vi "Get Message.vi"(8 "error in (no error)":errorcluster, 11 "SPARC4_GUI in":refnum<class "SPARC4_GUI.lvclass">) -> (0 "error out":errorcluster, 3 "SPARC4_GUI out":refnum<class "SPARC4_GUI.lvclass">)   [LabVIEW 2018, in "SPARC4_GUI.lvclass"]
uses:
  SPARC4_GUI.lvclass
  SPARC4_GUI.lvclass/SPARC4_GUI.ctl
  Channel GUI/Channel GUI.lvclass/Channel GUI.ctl
  Stream/Stream.lvclass
  Channel GUI/Channel GUI.lvclass
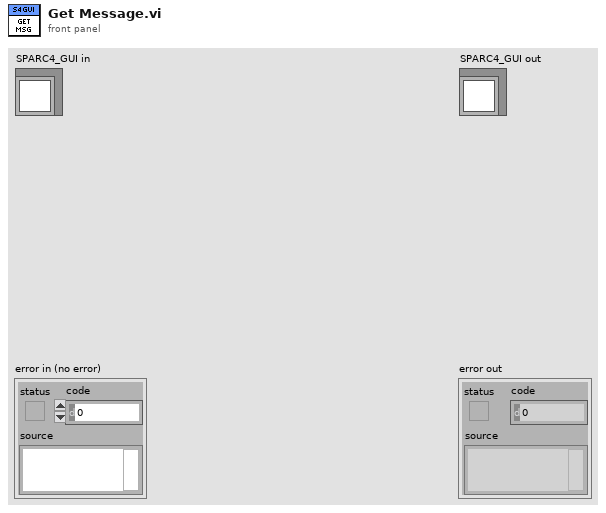
[diagram p1: front panel]
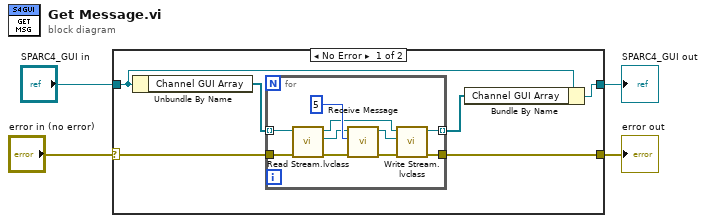
[diagram p0: block diagram]
diagram:
  n1 = case shown="No Error" "error in (no error)" {
    selector: "error in (no error)" -> [w6 w22]
    tunnel: [w8 w22] -> w3
    tunnel: [w9 w21] -> w1
    tunnel: "SPARC4_GUI in" -> [w10 w21]
    frame No Error {
      n2 = Unbundle By Name(w10) -> ("Channel GUI Array"=w7:refnum<class "Channel GUI.lvclass">[])
      n3 = for {
        tunnel: [w17] -> w8
        tunnel: w7 -> [w13] mode=indexing
        tunnel: w6 -> [w12]
        tunnel: [w11] -> w5 mode=indexing
        n4 = call "Read Stream.lvclass.vi"("error in (no error)"=w12, "Channel GUI in"=w13) -> ("error out"=w16:errorcluster, "Stream.lvclass"=w15:refnum<class "Stream.lvclass">, "Channel GUI out"=w14:refnum<class "Channel GUI.lvclass">)  [unwired: 7 in]
        n5 = call "Receive Message.vi"("error in (no error)"=w16, "timeout ms"=5, "Stream in"=w15) -> ("error out"=w19:errorcluster, "Stream out"=w18:refnum<class "Stream.lvclass">)  [unwired: 7 in]
        n6 = call "Write Stream.lvclass.vi"("error in (no error)"=w19, "Stream.lvclass"=w18, "Channel GUI in"=w14) -> ("error out"=w17:errorcluster, "Channel GUI out"=w11:refnum<class "Channel GUI.lvclass">)  [unwired: 7 in]
      }
      n7 = Bundle By Name(cluster=w10, "Channel GUI Array"=w5) -> (w9:refnum<class "SPARC4_GUI.lvclass">)
    }
    frame Error {
    }
  }
  "error out" <- w3
  "SPARC4_GUI out" <- w1
